vi "Client State Callback.vi"(7 "Owner":refnum<class>, 8 "error in (no error)":errorcluster, 10 "Connection State":T1, 11 "Connection":refnum<class "Connection.lvclass">) -> (0 "error out":errorcluster)   [LabVIEW 2020, in "Chat Client.lvclass"]
uses:
  Chat Client.lvclass
  lv-stream/stream/Connection/Connection.lvclass
  lv-stream/stream/Connection State.ctl
  Chat Client.lvclass/Chat Client.ctl
  Read Loop Async.vi
  lv-stream/stream/Stream.lvlib
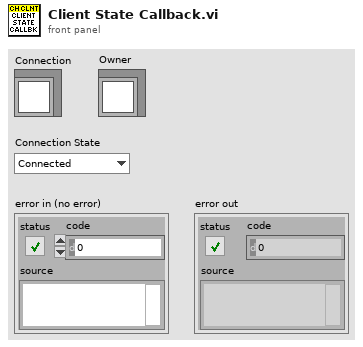
[diagram p1: front panel]
types:
  T1 = typedef "Stream.lvlib/Connection State.ctl" = enum16{"Connected", "Disconnected"}
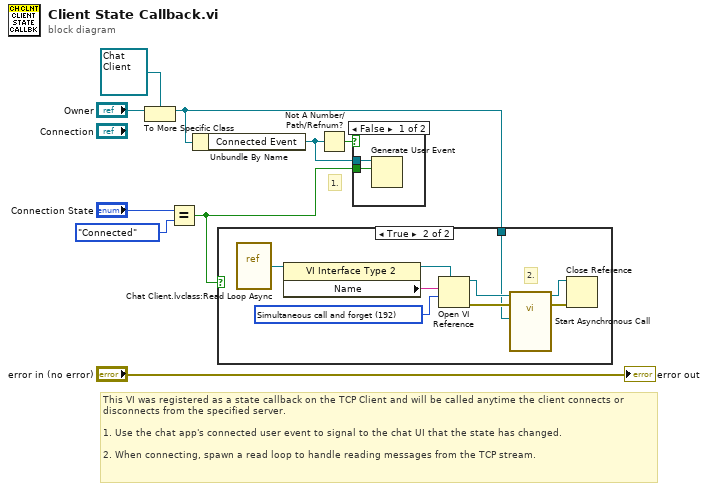
[diagram p0: block diagram]
diagram:
  # "This VI was registered as a state callback on the TCP Client and will be called anytime the client connects or disconnects from the specified server.\n\n1. Use the chat app's connected user event to signal to the chat UI that the state has changed.\n\n2. When connecting, spawn a read loop to handle reading messages from the TCP stream."
  # "1."
  n1 = To More Specific Class(target class=refnum<class "Chat Client.lvclass"> refnum ("Stream-TCP.lvlib:Chat Client.lvclass"), reference="Owner") -> (specific class reference=w4:refnum<class "Chat Client.lvclass">)  [unwired: 1 in, 1 out]
  n2 = Equal?(x="Connection State", y=Connection_State."Connected") -> (x = y?=w3:bool)
  n3 = Unbundle By Name(w4) -> ("Connected Event"=w2:refnum<user-event>)
  n4 = case shown="True" w3 {
    tunnel: w4 -> [_ w10]
    frame False {
    }
    frame True {
      w13 = 192 items=["Record modifications"=1, "Open templates for editing"=2, "Prompt user to save"=4, "Prepare for reentrant run"=8, "Prompt to find missing subVIs"=16, "Hide loading dialog box"=32, "Enable simultaneous calls"=64, "Prepare to call and forget"=128, "Simultaneous call and forget"=192, "Prepare to call and collect"=256, "Simultaneous call and collect"=320]
      # "2."
      n5 = vi-ref "Chat Client.lvclass:Read Loop Async.vi"() -> (w11:refnum<vi>)
      n6 = property class="VI Interface Type 2"(reference=w11) -> (reference out=w14:refnum<vi>, "Name"=w12:string)  [unwired: 1 in, 1 out]
      n7 = Open VI Reference(type specifier VI Refnum (for type only)=w14, vi path=w12, options=w13) -> (vi reference=w16:refnum<vi>, error out=w15:errorcluster)  [unwired: 3 in]
      n8 = call-by-ref "Start Asynchronous Call"(reference=w16, error in=w15, "Chat Client in"=w10) -> (reference out=w18:refnum<vi>, error out=w17:errorcluster)  [unwired: 11 in]
      n9 = Close Reference(reference=w18, error in (no error)=w17) -> ()  [unwired: 1 out]
    }
  }
  n10 = Not A Number/Path/Refnum?(number/path/refnum=w2) -> (NaN/Path/Refnum?=w1:bool)
  n11 = case shown="False" w1 {
    tunnel: w3 -> [w20 _]
    tunnel: w2 -> [w19 _]
    frame False {
      n12 = Generate User Event(user event=w19, event data cluster=w20) -> ()  [unwired: 2 in, 2 out]
    }
    frame True {
    }
  }
  "error out" <- "error in (no error)"
